vi "create.ModifyOrderShort.vi"(8 "error in (no error)":errorcluster, 11 "ModifyOrderShort.Parameters":T1={"Time Offset"=447000, "Order Id"="ORID0001", "Quantity"=20000, "Price"=1, "Modify Flags"=1}) -> (0 "error out":errorcluster, 2 "Bytes.out":u8[](array[numeric]) format="%.0x", 3 "MessageBase out":refnum<class "ModifyOrderShort.lvclass">)   [LabVIEW 2022 SP3]
uses:
  ModifyOrder/ModifyOrderShort.Parameters.ctl
  ModifyOrder/ModifyOrderShort.lvclass
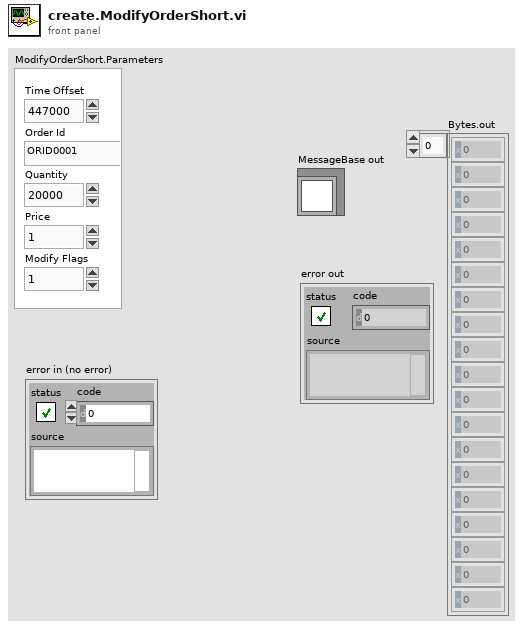
[diagram p1: front panel]
types:
  T1 = typedef "ModifyOrderShort.lvclass/ModifyOrderShort.Parameters.ctl" = cluster{"Time Offset":u32, "Order Id":string, "Quantity":u32, "Price":u16, "Modify Flags":u8}
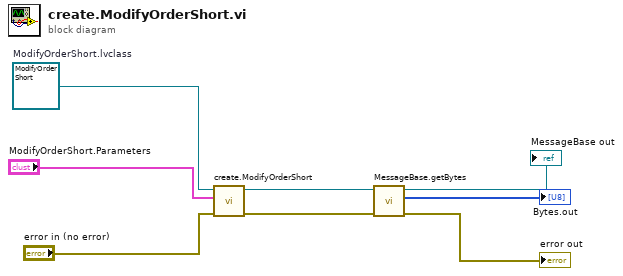
[diagram p0: block diagram]
diagram:
  w3 = refnum<class "ModifyOrderShort.lvclass"> refnum  # ModifyOrderShort.lvclass
  n1 = call-dynamic "create.ModifyOrderShort.vi"("error in"="error in (no error)", "ModifyOrderShort.Parameters"="ModifyOrderShort.Parameters", "ModifyOrderShort in"=w3) -> ("error out"=w6:errorcluster, "ModifyOrderShort out"=w7:refnum<class "ModifyOrderShort.lvclass">)  [unwired: 7 in]
  n2 = call-dynamic "MessageBase.getBytes.vi"("error in (no error)"=w6, "MessageBase in"=w7) -> ("error out"=→"error out":errorcluster, "Bytes.out"=→"Bytes.out":u8[], "MessageBase out"=→"MessageBase out":refnum<class "ModifyOrderShort.lvclass">)  [unwired: 7 in]
